vi "rs3 get sensor info.vi"(8 "error in (no error)":errorcluster, 10 "RS Camera info":u16(ring) items=["    RS2_CAMERA_INFO_NAME                           , /**< Friendly name */", "    RS2_CAMERA_INFO_SERIAL_NUMBER                  , /**< Device serial number */", "    RS2_CAMERA_INFO_FIRMWARE_VERSION               , /**< Primary firmware version */", "    RS2_CAMERA_INFO_PHYSICAL_PORT                       , /**< Unique identifier of the port the device is connected to (platform specific) */", "    RS2_CAMERA_INFO_DEBUG_OP_CODE                  , /**< If device supports firmware logging, this is the command to send to get logs from firmware */", "    RS2_CAMERA_INFO_ADVANCED_MODE                  , /**< True iff the device is in advanced mode */", "    RS2_CAMERA_INFO_PRODUCT_ID                     , /**< Product ID as reported in the USB descriptor */", "    RS2_CAMERA_INFO_CAMERA_LOCKED                  , /**< True iff EEPROM is locked */", "    RS2_CAMERA_INFO_COUNT                            /**< Number of enumeration values. Not a valid input: intended to be used in for-loops. */"], 11 "Sensor in":u64) -> (0 "error out":errorcluster, 1 "error":u64, 2 "Sensor info":string, 3 "Sensor out":u64)   [LabVIEW 2023]
doc: "Retrieves the SENSOR INFO for a specific sensor, based on the selection of pull-down menu. \n\nINPUT:\nRS camera info Select the type of info you are looking for about the sensor\nSensor in Sensor input handle\n\nOUTPUT:\nSensor info String containing the sensor info requested."
panel:
  # "RS3 Get Sensor Info"
  # "(C) 2017 Intel Corp.,  AGJ"
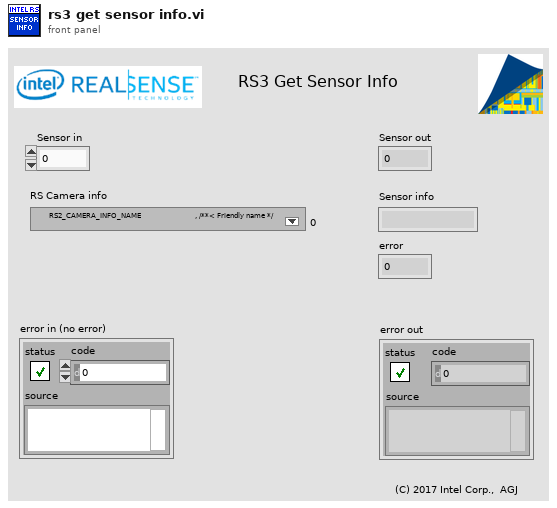
[diagram p1: front panel]
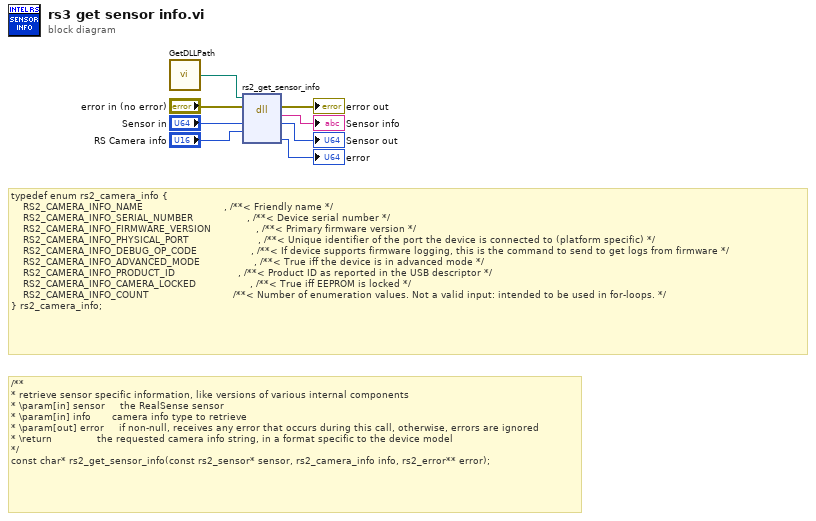
[diagram p0: block diagram]
diagram:
  # "/**\n* retrieve sensor specific information, like versions of various internal components\n* \\param[in] sensor     the RealSense sensor\n* \\param[in] info       camera info type to retrieve\n* \\param[out] error     if non-null, receives any error that occurs during this call, otherwise, errors are ignored\n* \\return               the requested camera info string, in a format specific to the device model\n*/\nconst char* rs2_get_sensor_info(const rs2_sensor* sensor, rs2_camera_info info, rs2_error** error);"
  # "typedef enum rs2_camera_info {\n    RS2_CAMERA_INFO_NAME                           , /**< Friendly name */\n    RS2_CAMERA_INFO_SERIAL_NUMBER                  , /**< Device serial number */\n    RS2_CAMERA_INFO_FIRMWARE_VERSION               , /**< Primary firmware version */\n    RS2_CAMERA_INFO_PHYSICAL_PORT                       , /**< Unique identifier of the port the device is connected to (platform specific) */\n    RS2_CAMERA_INFO_DEBUG_OP_CODE                  , /**< If device supports firmware logging, this is the command to send to get logs from firmware */\n    RS2_CAMERA_INFO_ADVANCED_MODE                  , /**< True iff the device is in advanced mode */\n    RS2_CAMERA_INFO_PRODUCT_ID                     , /**< Product ID as reported in the USB descriptor */\n    RS2_CAMERA_INFO_CAMERA_LOCKED                  , /**< True iff EEPROM is locked */\n    RS2_CAMERA_INFO_COUNT                            /**< Number of enumeration values. Not a valid input: intended to be used in for-loops. */\n} rs2_camera_info;"
  n1 = call "GetDLLPath.vi"() -> ("DLL Path"=w1:path)
  n2 = dll-call lib="C:/STEAMSyndicate/RealSenseWrappers/VI Wrappers (add ons) Public/RealSense/realsense2.dll" fn="rs2_get_sensor_info"(path in=w1, error in="error in (no error)", "sensor"="Sensor in", "info input"="RS Camera info") -> (error out=→"error out":errorcluster, "Sensor info output"=→"Sensor info":string, "sensor"=→"Sensor out":u64, "error"=→"error":u64)  [unwired: 3 in, 1 out]
